vi "Init TCP.vi"(8 "error in (no error)":errorcluster, 11 "Vecto in":refnum<class "Vecto.lvclass">) -> (0 "error out":errorcluster, 3 "Vecto out":refnum<class "Vecto.lvclass">)   [LabVIEW 2020, in "Vecto.lvlib" / "Vecto.lvclass"]
uses:
  Vecto.lvclass
  Vecto.lvclass/Vecto.ctl
  Node Config/Node Config.lvclass/Node Config.ctl
  proto/TcpClientHello/Data.ctl
  proto/TcpClientInfo/Data.ctl
  VectoTCPConnectionHandler/VectoTCPConnectionHandler.lvclass
  C:/dev/lv20CE/relink/lv-vecto/Vecto/TCPConnectionHandler/TCPConnectionHandler.lvclass
  Node Config/Node Config.lvclass
  TCPMessaging/TCPMessaging.lvclass
  proto/TcpClientHello/TcpClientHello.lvlib
  proto/TcpClientInfo/TcpClientInfo.lvlib
  IP Resolver/IP Resolver.lvclass
  IP Resolver/IP Target.ctl
  C:/dev/lv20CE/relink/lv-vecto/Vecto/VectoTCPConnectionHandler/VectoTCPConnectionHandler.lvclass
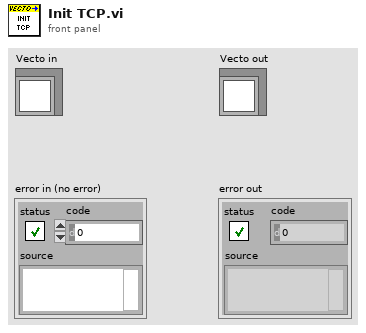
[diagram p1: front panel]
types:
  T1 = typedef "TcpClientHello.lvlib/Data.ctl" = cluster{"node_id":u32, "system":string, "cluster":string, "node_name":string, "app_version":string, "config_version":string, "config_hash":string, "node_alias":string}
  T2 = typedef "Vecto.lvlib/IP Resolver.lvclass/IP Target.ctl" = enum16{"Local", "External"}
  T3 = typedef "TcpClientInfo.lvlib/Data.ctl" = cluster{"node_id":u32, "node_name":string, "app_version":string, "config_version":string, "config_hash":string, "node_alias":string, "address":string}
  T4 = typedef "VectoConfig.lvlib/Node Info.ctl" = cluster{"System":string, "Cluster":string, "Name":string, "ID":u32, "Capabilities":string[]}
  T5 = typedef "VectoConfig.lvlib/TCP Messaging Info.ctl" = cluster{"Address":string, "Port":u16, "Server (Client)":bool}
  T6 = typedef "VectoConfig.lvlib/Target Group Info.ctl" = cluster{"Name":string, "ID":u32, "Nodes":T7[]}
  T7 = typedef "VectoConfig.lvlib/Node Name ID.ctl" = cluster{"Name":string, "ID":u32}
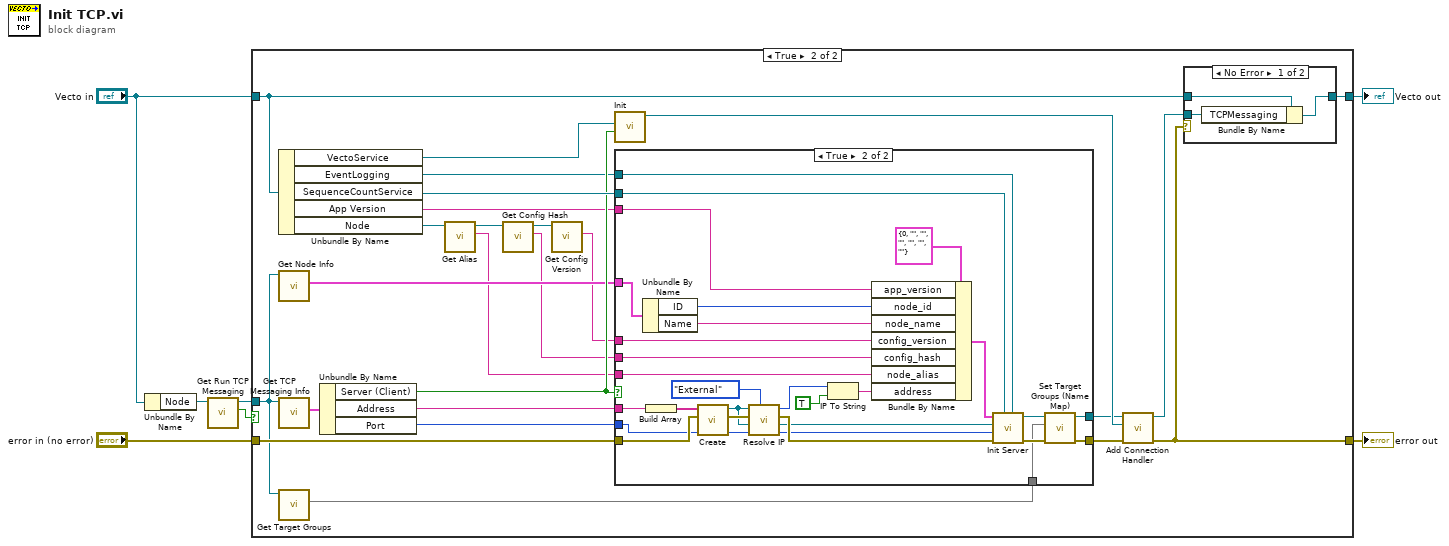
[diagram p0: block diagram]
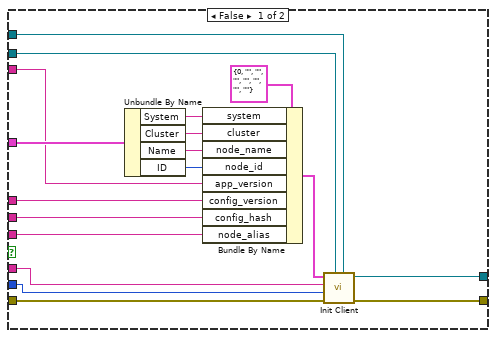
[diagram p3: hidden frame]
diagram:
  n1 = Unbundle By Name("Vecto in") -> ("Node"=w7:refnum<class "Node Config.lvclass">)
  n2 = call "Get Run TCP Messaging.vi"("Node Config in"=w7) -> ("Run TCP Messaging"=w6:bool, "Node Config out"=w4:refnum<class "Node Config.lvclass">)  [unwired: 8 in, 1 out]
  n3 = case shown="True" w6 {
    tunnel: "error in (no error)" -> [w8 w34]
    tunnel: w4 -> [_ w10]
    tunnel: "Vecto in" -> [w9 w29]
    tunnel: [w8 w25] -> w2
    tunnel: [w9 w28] -> w1
    frame False {
    }
    frame True {
      n4 = Unbundle By Name(w29) -> ("VectoService"=w27:refnum<class "VectoInfo.lvclass">, "EventLogging"=w20:refnum<class "EventLoggingService.lvclass">, "SequenceCountService"=w30:refnum<class "SequenceCountService.lvclass">, "App Version"=w21:string, "Node"=w16:refnum<class "Node Config.lvclass">)
      n5 = call "Get Node Info.vi"("Node Config in"=w10) -> ("Info"=w22:T4)  [unwired: 8 in, 2 out]
      n6 = call "Get TCP Messaging Info.vi"("Node Config in"=w10) -> ("TCP Messaging Info"=w33:T5)  [unwired: 8 in, 2 out]
      n7 = call "Get Target Groups.vi"("Node Config in"=w10) -> ("Target Groups"=w19:map{string, T6})  [unwired: 8 in, 2 out]
      n8 = Unbundle By Name(w33) -> ("Server (Client)"=w26:bool, "Address"=w32:string, "Port"=w31:u16)
      n9 = call "Get Alias.vi"("Node Config in"=w16) -> ("Node Alias"=w11:string, "Node Config out"=w12:refnum<class "Node Config.lvclass">)  [unwired: 8 in, 1 out]
      n10 = call "Get Config Hash.vi"("Node Config in"=w12) -> ("Config Hash"=w14:string, "Node Config out"=w15:refnum<class "Node Config.lvclass">)  [unwired: 8 in, 1 out]
      n11 = call "Get Config Version.vi"("Node Config in"=w15) -> ("Config Version"=w13:string)  [unwired: 8 in, 2 out]
      n12 = call "Init.vi"("Server (Client)"=w26, "VectoInfo"=w27) -> ("VectoTCPConnectionHandler out"=w23:refnum<class "VectoTCPConnectionHandler.lvclass">)  [unwired: 8 in, 1 out]
      n13 = case shown="True" w26 {
        tunnel: w34 -> [w52 w78]
        tunnel: w32 -> [w42 w60]
        tunnel: w31 -> [w41 w77]
        tunnel: w30 -> [w49 w76]
        tunnel: [w50 w70] -> w18
        tunnel: [w51 w69] -> w17
        tunnel: w22 -> [w46 w75]
        tunnel: w21 -> [w40 w61]
        tunnel: w20 -> [w38 w74]
        tunnel: w19 -> [_ w72]
        tunnel: w14 -> [w37 w64]
        tunnel: w13 -> [w36 w65]
        tunnel: w11 -> [w35 w63]
        frame False {
          n14 = Unbundle By Name(w46) -> ("System"=w45:string, "Cluster"=w44:string, "Name"=w43:string, "ID"=w39:u32)
          n15 = Bundle By Name(cluster=T1 {"node_id"=0, "system"="", "cluster"="", "node_name"="", "app_version"="", "config_version"="", "config_hash"="", "node_alias"=""} ("Client Info"), "system"=w45, "cluster"=w44, "node_name"=w43, "node_id"=w39, "app_version"=w40, "config_version"=w36, "config_hash"=w37, "node_alias"=w35) -> (w47:T1)
          n16 = call "Init Client.vi"("EventLogger"=w38, "SequenceCountService"=w49, "error in (no error)"=w52, "Remote Port"=w41, "Remote Address"=w42, "Client Info"=w47) -> ("error out"=w51:errorcluster, "TCPMessaging out"=w50:refnum<class "TCPMessaging.lvclass">)  [unwired: 4 in]
        }
        frame True {
          n17 = Unbundle By Name(w75) -> ("ID"=w66:u32, "Name"=w62:string)
          n18 = Build Array(w60) -> (w59:string[])
          n19 = call "Create.vi"("error in (no error)"=w78, "Bindings"=w59) -> ("error out"=w58:errorcluster, "IP Resolver"=w53:refnum<class "IP Resolver.lvclass">)  [unwired: 8 in]
          n20 = call "Resolve IP.vi"("IP Target (Local)"=IP_Target."External", "error in (no error)"=w58, "IP Resolver in"=w53) -> ("error out"=w79:errorcluster, "U32 Address"=w56:u32)  [unwired: 7 in]
          n21 = IP To String(1:TRUE ("dot notation? (F)"), 2:w56) -> (0:w54:string)
          n22 = Bundle By Name(cluster=T3 {"node_id"=0, "node_name"="", "app_version"="", "config_version"="", "config_hash"="", "node_alias"="", "address"=""} ("Server Info"), "app_version"=w61, "node_id"=w66, "node_name"=w62, "config_version"=w65, "config_hash"=w64, "node_alias"=w63, "address"=w54) -> (w67:T3)
          n23 = call "Init Server.vi"("EventLogger"=w74, "SequenceCountService"=w76, "error in (no error)"=w79, "Bind Port"=w77, "IP Resolver"=w53, "Server Info"=w67) -> ("error out"=w73:errorcluster, "TCPMessaging out"=w71:refnum<class "TCPMessaging.lvclass">)  [unwired: 4 in]
          n24 = call "Set Target Groups (Name Map).vi"("error in (no error)"=w73, "Target Groups"=w72, "TCPMessaging in"=w71) -> ("error out"=w69:errorcluster, "TCPMessaging out"=w70:refnum<class "TCPMessaging.lvclass">)  [unwired: 7 in]
        }
      }
      n25 = call "Add Connection Handler.vi"("error in (no error)"=w17, "TCPConnectionHandler"=w23, "TCPMessaging in"=w18) -> ("error out"=w25:errorcluster, "TCPMessaging out"=w24:refnum<class "TCPMessaging.lvclass">)  [unwired: 7 in]
      n26 = case shown="No Error" w25 {
        tunnel: w29 -> [w82 w83]
        tunnel: w24 -> [w81 _]
        tunnel: [w80 w83] -> w28
        frame No Error {
          n27 = Bundle By Name(cluster=w82, "TCPMessaging"=w81) -> (w80:refnum<class "Vecto.lvclass">)
        }
        frame Error {
        }
      }
    }
  }
  "error out" <- w2
  "Vecto out" <- w1
